vi "uc480_SubVI_Example_Init_Camera_Error_Handling.vi"(8 "Error In":errorcluster, 11 ".NET (Reference)":refnum<k24>) -> (0 "Error Out":errorcluster)   [LabVIEW 2016]
uses:
  D:/Fabrizio/Labview Projects/IR OPO Controller/Branches/Final version/uc480DotNet.dll
  uc480DotNet.dll
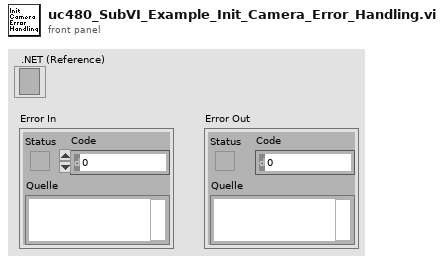
[diagram p1: front panel]
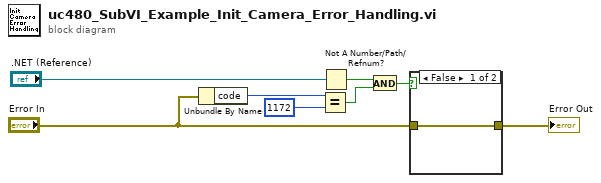
[diagram p0: block diagram]
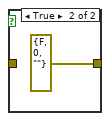
[diagram p2: hidden frame]
diagram:
  n1 = Unbundle By Name("Error In") -> ("code"=w2:i32)
  n2 = Equal?(x=w2, y=1172) -> (x = y?=w5:bool)
  n3 = Not A Number/Path/Refnum?(number/path/refnum=".NET (Reference)") -> (NaN/Path/Refnum?=w4:bool)
  n4 = And(x=w4, y=w5) -> (x .and. y?=w6:bool)
  n5 = case shown="False" w6 {
    tunnel: "Error In" -> [w9 _]
    tunnel: [w9 errorcluster {"status"=FALSE, "code"=0, "source"=""} ("Error Out")] -> w8
    frame False {
    }
    frame True {
    }
  }
  "Error Out" <- w8
